vi "constructor.vi"(8 "error in (no error)":errorcluster, 9 "machine name":string, 10 "Camera":string) -> (0 "error out":errorcluster, 3 "NetworkCamera out":refnum<class "NetworkCamera.lvclass">)   [LabVIEW 2009, in "Hardware.lvlib" / "HWControllers.lvlib" / "NetworkCamera.lvclass"]
uses:
  NetworkCamera.lvclass
  Tools/Filing/FileSystem/FileSystem.lvclass
  NetworkPixelfly/NetworkPixelfly.lvclass
  Channels/Camera/PixelflySA/PixelflySA.lvclass
  NetworkCamera.lvclass/NetworkCamera.ctl
  Channels/Camera/Camera/Camera.lvclass
  Channels/Camera/ProEM_WinX32/ProEM_WinX32.lvclass
  Network_ProEM_WinX32/Network_ProEm_WinX32/Network_ProEm_WinX32.lvclass
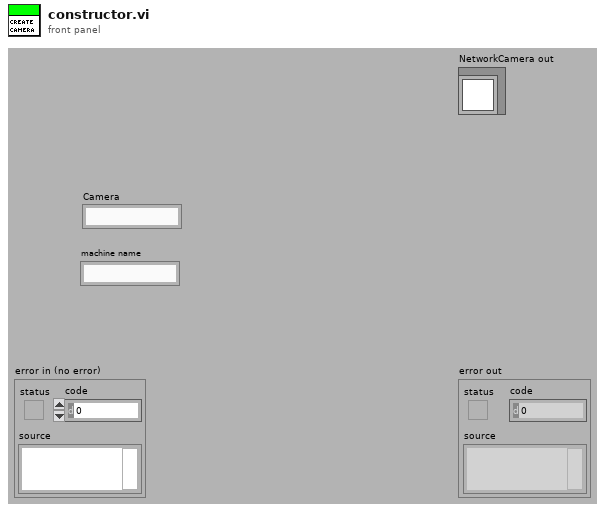
[diagram p1: front panel]
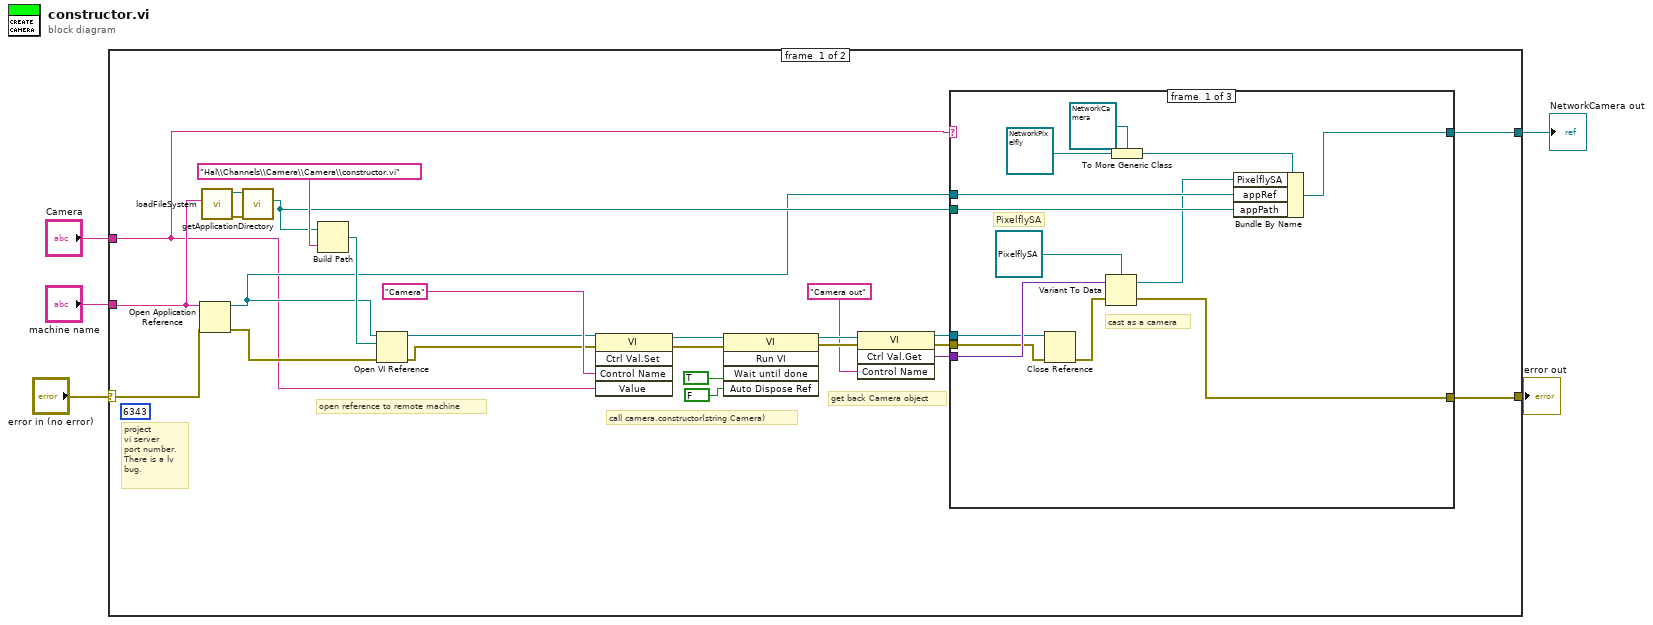
[diagram p0: block diagram]
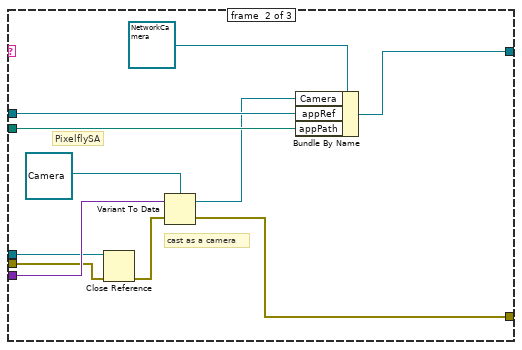
[diagram p2: hidden frame]
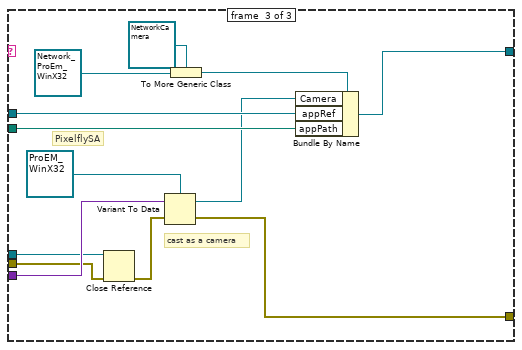
[diagram p3: hidden frame]
diagram:
  n1 = case shown="No Error" "error in (no error)" {
    selector: "error in (no error)" -> [w30 w68]
    tunnel: [w13 w68] -> w4
    tunnel: [w12 _] -> w3
    tunnel: "Camera" -> [w6 _]
    tunnel: "machine name" -> [w29 _]
    frame #0 {
      (unwired) u16 6343 ("port number or service name (3363)")
      # "project \nvi server \nport number.\nThere is a lv\nbug."
      # "open reference to remote machine"
      # "get back Camera object"
      # "call camera.constructor(string Camera)"
      n2 = Open Application Reference(8:w30, 11:w29) -> (0:w24:errorcluster, 3:w7:refnum<vi>)  [unwired: 2 in]
      n3 = call "loadFileSystem.vi"("computer name"=w29) -> ("error out"=w27:errorcluster, "FileSystem out"=w28:refnum<class "FileSystem.lvclass">)  [unwired: 9 in]
      n4 = call-dynamic "getApplicationDirectory.vi"("error in (no error)"=w27, "FileSystem.lvclass in"=w28) -> ("ApplicationDirectory"=w11:path)  [unwired: 7 in, 2 out]
      n5 = Build Path(base path=w11, name or relative path="Hal\\Channels\\Camera\\Camera\\constructor.vi") -> (appended path=w25:path)
      n6 = Open VI Reference(application reference (local)=w7, vi path=w25, error in (no error)=w24) -> (vi reference=w10:refnum<vi>, error out=w9:errorcluster)  [unwired: 3 in]
      n7 = invoke class="VI" method="Ctrl Val.Set"(reference=w10, error in=w9, "Control Name"="Camera", "Value"=w6) -> (reference out=w22:refnum<vi>, error out=w21:errorcluster)  [unwired: 1 in, 3 out]
      n8 = invoke class="VI" method="Run VI"(reference=w22, error in=w21, "Wait until done"=TRUE, "Auto Dispose Ref"=FALSE) -> (reference out=w19:refnum<vi>, error out=w18:errorcluster)  [unwired: 1 in, 3 out]
      n9 = invoke class="VI" method="Ctrl Val.Get"(reference=w19, error in=w18, "Control Name"="Camera out") -> (reference out=w14:refnum<vi>, error out=w15:errorcluster, "Get Control Value Variant"=w16:variant)  [unwired: 1 in, 1 out]
      n10 = case shown="Default" w6 {
        tunnel: w16 -> [w43 w54 w67]
        tunnel: w15 -> [w42 w53 w66]
        tunnel: w14 -> [w41 w52 w65]
        tunnel: [w39 w50 w63] -> w13
        tunnel: [w38 w49 w62] -> w12
        tunnel: w11 -> [w37 w48 w61]
        tunnel: w7 -> [w36 w47 w60]
        frame #0 {
          # "PixelflySA"
          # "cast as a camera"
          n11 = Close Reference(reference=w41, error in (no error)=w42) -> (error out=w40:errorcluster)
          n12 = Variant To Data(error in=w40, Variant=w43, type=refnum<class "PixelflySA.lvclass"> refnum ("PixelflySA.lvclass")) -> (error out=w39:errorcluster, data=w35:refnum<class "PixelflySA.lvclass">)
          n13 = To More Generic Class(target class=refnum<class "NetworkCamera.lvclass"> refnum ("NetworkCamera out"), reference=refnum<class "NetworkPixelfly.lvclass"> refnum ("Hardware:HWControllers.lvlib:NetworkPixelfly.lvclass")) -> (generic class reference=w31:refnum<class "NetworkCamera.lvclass">)
          n14 = Bundle By Name(cluster=w31, "PixelflySA"=w35, "appRef"=w36, "appPath"=w37) -> (w38:refnum<class "NetworkCamera.lvclass">)
        }
        frame #1 {
          # "PixelflySA"
          # "cast as a camera"
          n15 = Close Reference(reference=w52, error in (no error)=w53) -> (error out=w51:errorcluster)
          n16 = Variant To Data(error in=w51, Variant=w54, type=refnum<class "Camera.lvclass"> refnum ("Hardware:Channels.lvlib:Camera.lvclass")) -> (error out=w50:errorcluster, data=w46:refnum<class "Camera.lvclass">)
          n17 = Bundle By Name(cluster=refnum<class "NetworkCamera.lvclass"> refnum ("NetworkCamera out"), "Camera"=w46, "appRef"=w47, "appPath"=w48) -> (w49:refnum<class "NetworkCamera.lvclass">)
        }
        frame #2 {
          # "PixelflySA"
          # "cast as a camera"
          n18 = Close Reference(reference=w65, error in (no error)=w66) -> (error out=w64:errorcluster)
          n19 = Variant To Data(error in=w64, Variant=w67, type=refnum<class "ProEM_WinX32.lvclass"> refnum ("Hardware:Channels.lvlib:ProEM_WinX32.lvclass")) -> (error out=w63:errorcluster, data=w59:refnum<class "ProEM_WinX32.lvclass">)
          n20 = To More Generic Class(target class=refnum<class "NetworkCamera.lvclass"> refnum ("NetworkCamera out"), reference=refnum<class "Network_ProEm_WinX32.lvclass"> refnum ("Hardware:HWControllers.lvlib:Network_ProEm_WinX32.lvclass")) -> (generic class reference=w57:refnum<class "NetworkCamera.lvclass">)
          n21 = Bundle By Name(cluster=w57, "Camera"=w59, "appRef"=w60, "appPath"=w61) -> (w62:refnum<class "NetworkCamera.lvclass">)
        }
      }
    }
    frame #1 {
    }
  }
  "error out" <- w4
  "NetworkCamera out" <- w3
